vi "SetHomeOffset.vi"(8 "error in (no error)":errorcluster, 10 "Offset":dbl, 11 "ThorlabsLabJack in":refnum<class "ThorlabsLabJack.lvclass">) -> (0 "error out":errorcluster, 3 "ThorlabsLabJack out":refnum<class "ThorlabsLabJack.lvclass">)   [LabVIEW 2018, in "ThorlabsLabJack.lvlib" / "ThorlabsLabJack.lvclass"]
uses:
  ThorlabsLabJack.lvclass
  ThorlabsLabJack.lvclass/ThorlabsLabJack.ctl
  C:/Projects/LabVIEW/In-Progress/Chetan Malpure/Axis/Thorlabs LabJack/Drivers/Thorlabs.MotionControl.IntegratedStepperMotorsCLI.dll
  Drivers/Thorlabs.MotionControl.IntegratedStepperMotorsCLI.dll
  C:/Projects/LabVIEW/In-Progress/Chetan Malpure/Axis/Thorlabs LabJack/Drivers/Thorlabs.MotionControl.GenericMotorCLI.dll
  Drivers/Thorlabs.MotionControl.GenericMotorCLI.dll
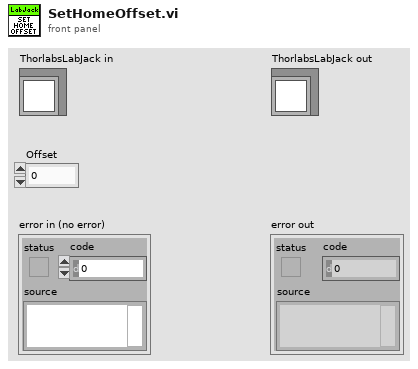
[diagram p1: front panel]
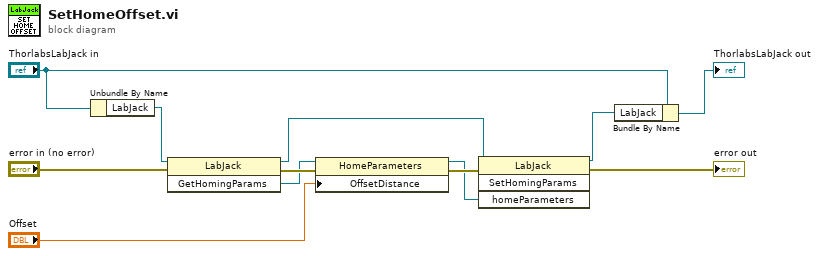
[diagram p0: block diagram]
diagram:
  n1 = Unbundle By Name("ThorlabsLabJack in") -> ("LabJack"=w8:refnum<k24>)
  n2 = invoke class="LabJack" method="GetHomingParams"(reference=w8, error in="error in (no error)") -> (reference out=w4:refnum<k24>, error out=w6:errorcluster, "GetHomingParams"=w2:refnum<k24>)  [unwired: 1 in]
  n3 = property class="HomeParameters"(reference=w2, error in=w6, "OffsetDistance"="Offset") -> (reference out=w1:refnum<k24>, error out=w3:errorcluster)
  n4 = invoke class="LabJack" method="SetHomingParams"(reference=w4, error in=w3, "homeParameters"=w1) -> (reference out=w9:refnum<k24>, error out=→"error out":errorcluster)  [unwired: 1 in, 2 out]
  n5 = Bundle By Name(cluster="ThorlabsLabJack in", "LabJack"=w9) -> (→"ThorlabsLabJack out":refnum<class "ThorlabsLabJack.lvclass">)
